vi "Close DAQ.vi"(8 "error in (no error)":errorcluster, 11 "Refnum in":refnum<k21>) -> ()   [LabVIEW 2016]
uses:
  <vilib>/Utility/error.llb/DialogType.ctl
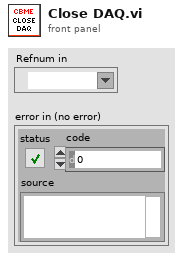
[diagram p1: front panel]
types:
  T1 = typedef "DialogType.ctl" = u16
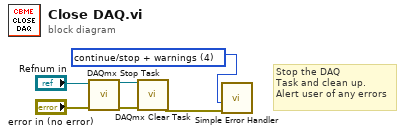
[diagram p0: block diagram]
diagram:
  w4 = T1 4 items=["no dialog", "OK message", "continue or stop message", "OK message + warnings", "continue/stop + warnings"] ("type of dialog (OK msg:1)")
  # "Stop the DAQ \nTask and clean up.\nAlert user of any errors"
  n1 = call <vilib>:"DAQmx Stop Task.vi"("task/channels in"="Refnum in", "error in"="error in (no error)") -> ("task out"=w1:refnum<k21>, "error out"=w2:errorcluster)  [unwired: 12 in]
  n2 = call <vilib>:"DAQmx Clear Task.vi"("task in"=w1, "error in"=w2) -> ("error out"=w3:errorcluster)  [unwired: 13 in]
  n3 = call <vilib>:"Simple Error Handler.vi"("type of dialog (OK msg:1)"=w4, "error in (no error)"=w3) -> ()  [unwired: 3 in, 5 out]
